vi "SVT Set Swept Sine Propagation Delays.vi"(8 "error in (no error)":errorcluster, 9 "DUT propagation time [ms]":dbl format="%.2f", 10 "device propagation delay [samples]":dbl=1.0 format="%#.1g", 11 "swept sine task in":T1={"source settings"={"AO task name"="", "source"=[]}, "stimulus settings"={"stimulus task name"="", "stimulus"=[]}, "response(s) settings"={"response task name"="", "response"=[]}, "measurement settings"={"AI sampling frequency"=51200.0, "AO sampling frequency"=51200.0, "AI block size"=5120, "AO block Size"=5120, "block duration [ms]"=100.0, "number of AI channels"=0, "device propagation delay [samples]"=1.0, "total propagation time [samples]"=0.0, "DUT propagation time [ms]"=0.0}, "linlog"=enum."linear", "repeat"=enum."off", "frequency list"=[500.0, 515.1515151515151, 530.3030303030303, 545.4545454545454, 560.6060606060605, 575.7575757575756, 590.9090909090908, 606.0606060606059, 621.212121212121, 636.3636363636361, 651.5151515151513, 666.6666666666664, 681.8181818181815, 696.9696969696967, 712.1212121212118, 727.2727272727269, 742.424242424242, 757.5757575757572, 772.7272727272723, 787.8787878787874, 803.0303030303025, 818.1818181818177, 833.3333333333328, 848.4848484848479, 863.6363636363631, 878.7878787878782, 893.9393939393933, 909.0909090909084, 924.2424242424236, 939.3939393939387, 954.5454545454538, 969.696969696969, 984.8484848484841, 999.9999999999992, 1015.1515151515143, 1030.3030303030296, 1045.4545454545448, 1060.60606060606, 1075.7575757575753, 1090.9090909090905, 1106.0606060606058, 1121.212121212121, 1136.3636363636363, 1151.5151515151515, 1166.6666666666667, 1181.818181818182, 1196.9696969696972, 1212.1212121212125, 1227.2727272727277, 1242.424242424243, 1257.5757575757582, 1272.7272727272734, 1287.8787878787887, 1303.030303030304, 1318.1818181818192, 1333.3333333333344, 1348.4848484848496, 1363.6363636363649, 1378.7878787878801, 1393.9393939393954, 1409.0909090909106, 1424.2424242424258, 1439.393939393941, 1454.5454545454563, 1469.6969696969716, 1484.8484848484868, 1500.000000000002, 1515.1515151515173, 1530.3030303030325, 1545.4545454545478, 1560.606060606063, 1575.7575757575783, 1590.9090909090935, 1606.0606060606087, 1621.212121212124, 1636.3636363636392, 1651.5151515151545, 1666.6666666666697, 1681.818181818185, 1696.9696969697002, 1712.1212121212154, 1727.2727272727307, 1742.424242424246, 1757.5757575757611, 1772.7272727272764, 1787.8787878787916, 1803.0303030303069, 1818.181818181822, 1833.3333333333374, 1848.4848484848526, 1863.6363636363678, 1878.787878787883, 1893.9393939393983, 1909.0909090909136, 1924.2424242424288, 1939.393939393944, 1954.5454545454593, 1969.6969696969745, 1984.8484848484898, 2000.000000000005], "amplitude list"=[1.0, 1.0, 1.0, 1.0, 1.0, 1.0, 1.0, 1.0, 1.0, 1.0, 1.0, 1.0, 1.0, 1.0, 1.0, 1.0, 1.0, 1.0, 1.0, 1.0, 1.0, 1.0, 1.0, 1.0, 1.0, 1.0, 1.0, 1.0, 1.0, 1.0, 1.0, 1.0, 1.0, 1.0, 1.0, 1.0, 1.0, 1.0, 1.0, 1.0, 1.0, 1.0, 1.0, 1.0, 1.0, 1.0, 1.0, 1.0, 1.0, 1.0, 1.0, 1.0, 1.0, 1.0, 1.0, 1.0, 1.0, 1.0, 1.0, 1.0, 1.0, 1.0, 1.0, 1.0, 1.0, 1.0, 1.0, 1.0, 1.0, 1.0, 1.0, 1.0, 1.0, 1.0, 1.0, 1.0, 1.0, 1.0, 1.0, 1.0, 1.0, 1.0, 1.0, 1.0, 1.0, 1.0, 1.0, 1.0, 1.0, 1.0, 1.0, 1.0, 1.0, 1.0, 1.0, 1.0, 1.0, 1.0, 1.0, 1.0], "settling time"={"settle time"=0.02, "settle cycles"=5}, "integration time"={"integration time"=0.02, "integration cycles"=5}, "frequencies indices"={"AI freq index"=0, "AO freq index"=0}, "read marks"={"write index"=0, "read index"=0, "freq start index"=0, "freq stop index"=0, "# extracted"=0, "buffer type"=enum."Invalid buffer", "read/write indices"=[{"settle time index"=0, "integration time index"=0}, {"settle time index"=0, "integration time index"=0}, {"settle time index"=0, "integration time index"=0}], "AO index"=0, "AI index"=0, "settled"=FALSE, "integration done"=FALSE}, "harmonic settings"={"maximum THD harmonic"=0, "harmonic mapping"=[], "units"={"THD unit"=enum."%", "nth harmonic unit"=enum."%", "SINAD unit"=enum."dB", "THD+N unit"=enum."dB"}}, "auto resolution settings"={"auto max step"=512, "slow threshold db"=6.0, "fast threshold db"=1.0}, "auto level settings"={"auto level enable"=FALSE, "auto level channel"=6, "ideal ref"=1.0, "max level"=10.0, "ref upper deviation db"=3.0, "ref lower deviation db"=-3.0}, "offset"=0.0, "ramping rate"=0.0, "phase"=0.0, "initialize"=FALSE} {"phase" format="%.2f"; "response(s) settings"."response"."channel info"."pregain" format="%.2f"; "response(s) settings"."response"."channel info"."weighting filter" items=["Linear", "A-weighting", "B-weighting", "C-weighting", "ITU-R 468-4", "Dolby", "CCITT", "C-message", "Wb", "Wc", "Wd", "We", "Wf", "Wh", "Wj", "Wk", "Wm", "AES17 20 kHz lowpass", "AES17 40 kHz lowpass", "AES17 20 kHz highpass", "AES17 40 kHz highpass"]; "response(s) settings"."response"."channel info"."dB reference" format="%^.1e"; "response(s) settings"."response"."channel info"."engineering units" items=["custom..."=0, "V"=1, "A"=21, "C"=30, "pC"=31, "s"=32, "-"=29, "Pa"=2, "N"=20, "g"=3, "m/s^2"=4, "m/s"=5, "m"=6, "mm/s"=12, "mm"=13, "micron/s"=14, "micron"=15, "in/s^2"=7, "in/s"=8, "in"=9, "mil/s"=10, "mil"=11, "rad/s^2"=16, "rad/s"=17, "rad"=18, "deg/s^2"=26, "deg/s"=27, "deg"=28, "RPM"=22, "cycle/s^2"=23, "Hz"=24, "cycle"=25, "strain"=19]; "response(s) settings"."response"."channel info"."sensor sensitivity" format="%#_5f"; "stimulus settings"."stimulus"."channel info"."pregain" format="%.2f"; "stimulus settings"."stimulus"."channel info"."weighting filter" items=["Linear", "A-weighting", "B-weighting", "C-weighting", "ITU-R 468-4", "Dolby", "CCITT", "C-message", "Wb", "Wc", "Wd", "We", "Wf", "Wh", "Wj", "Wk", "Wm", "AES17 20 kHz lowpass", "AES17 40 kHz lowpass", "AES17 20 kHz highpass", "AES17 40 kHz highpass"]; "stimulus settings"."stimulus"."channel info"."dB reference" format="%^.1e"; "stimulus settings"."stimulus"."channel info"."engineering units" items=["custom..."=0, "V"=1, "A"=21, "C"=30, "pC"=31, "s"=32, "-"=29, "Pa"=2, "N"=20, "g"=3, "m/s^2"=4, "m/s"=5, "m"=6, "mm/s"=12, "mm"=13, "micron/s"=14, "micron"=15, "in/s^2"=7, "in/s"=8, "in"=9, "mil/s"=10, "mil"=11, "rad/s^2"=16, "rad/s"=17, "rad"=18, "deg/s^2"=26, "deg/s"=27, "deg"=28, "RPM"=22, "cycle/s^2"=23, "Hz"=24, "cycle"=25, "strain"=19]; "stimulus settings"."stimulus"."channel info"."sensor sensitivity" format="%#_5f"; "ramping rate" format="%.4f"; "offset" format="%.2f"; "auto level settings"."ref lower deviation db" format="%.4f"; "auto level settings"."ref upper deviation db" format="%.4f"; "auto level settings"."max level" format="%.4f"; "auto level settings"."ideal ref" format="%.4f"; "auto resolution settings"."fast threshold db" format="%.4f"; "auto resolution settings"."slow threshold db" format="%.4f"; "harmonic settings"."maximum THD harmonic" max=10 step=1; "integration time"."integration time" format="%.2p"; "settling time"."settle time" format="%.2p"; "amplitude list" format="%.2f"; "frequency list" format="%.2f"; "measurement settings"."DUT propagation time [ms]" format="%.2f"; "measurement settings"."AO sampling frequency" format="%.2f"; "measurement settings"."AI sampling frequency" format="%.2f"}) -> (0 "error out":errorcluster, 3 "swept sine task out":T1={"source settings"={"AO task name"="", "source"=[]}, "stimulus settings"={"stimulus task name"="", "stimulus"=[]}, "response(s) settings"={"response task name"="", "response"=[]}, "measurement settings"={"AI sampling frequency"=51200.0, "AO sampling frequency"=51200.0, "AI block size"=5120, "AO block Size"=5120, "block duration [ms]"=100.0, "number of AI channels"=0, "device propagation delay [samples]"=1.0, "total propagation time [samples]"=0.0, "DUT propagation time [ms]"=0.0}, "linlog"=enum."linear", "repeat"=enum."off", "frequency list"=[500.0, 515.1515151515151, 530.3030303030303, 545.4545454545454, 560.6060606060605, 575.7575757575756, 590.9090909090908, 606.0606060606059, 621.212121212121, 636.3636363636361, 651.5151515151513, 666.6666666666664, 681.8181818181815, 696.9696969696967, 712.1212121212118, 727.2727272727269, 742.424242424242, 757.5757575757572, 772.7272727272723, 787.8787878787874, 803.0303030303025, 818.1818181818177, 833.3333333333328, 848.4848484848479, 863.6363636363631, 878.7878787878782, 893.9393939393933, 909.0909090909084, 924.2424242424236, 939.3939393939387, 954.5454545454538, 969.696969696969, 984.8484848484841, 999.9999999999992, 1015.1515151515143, 1030.3030303030296, 1045.4545454545448, 1060.60606060606, 1075.7575757575753, 1090.9090909090905, 1106.0606060606058, 1121.212121212121, 1136.3636363636363, 1151.5151515151515, 1166.6666666666667, 1181.818181818182, 1196.9696969696972, 1212.1212121212125, 1227.2727272727277, 1242.424242424243, 1257.5757575757582, 1272.7272727272734, 1287.8787878787887, 1303.030303030304, 1318.1818181818192, 1333.3333333333344, 1348.4848484848496, 1363.6363636363649, 1378.7878787878801, 1393.9393939393954, 1409.0909090909106, 1424.2424242424258, 1439.393939393941, 1454.5454545454563, 1469.6969696969716, 1484.8484848484868, 1500.000000000002, 1515.1515151515173, 1530.3030303030325, 1545.4545454545478, 1560.606060606063, 1575.7575757575783, 1590.9090909090935, 1606.0606060606087, 1621.212121212124, 1636.3636363636392, 1651.5151515151545, 1666.6666666666697, 1681.818181818185, 1696.9696969697002, 1712.1212121212154, 1727.2727272727307, 1742.424242424246, 1757.5757575757611, 1772.7272727272764, 1787.8787878787916, 1803.0303030303069, 1818.181818181822, 1833.3333333333374, 1848.4848484848526, 1863.6363636363678, 1878.787878787883, 1893.9393939393983, 1909.0909090909136, 1924.2424242424288, 1939.393939393944, 1954.5454545454593, 1969.6969696969745, 1984.8484848484898, 2000.000000000005], "amplitude list"=[1.0, 1.0, 1.0, 1.0, 1.0, 1.0, 1.0, 1.0, 1.0, 1.0, 1.0, 1.0, 1.0, 1.0, 1.0, 1.0, 1.0, 1.0, 1.0, 1.0, 1.0, 1.0, 1.0, 1.0, 1.0, 1.0, 1.0, 1.0, 1.0, 1.0, 1.0, 1.0, 1.0, 1.0, 1.0, 1.0, 1.0, 1.0, 1.0, 1.0, 1.0, 1.0, 1.0, 1.0, 1.0, 1.0, 1.0, 1.0, 1.0, 1.0, 1.0, 1.0, 1.0, 1.0, 1.0, 1.0, 1.0, 1.0, 1.0, 1.0, 1.0, 1.0, 1.0, 1.0, 1.0, 1.0, 1.0, 1.0, 1.0, 1.0, 1.0, 1.0, 1.0, 1.0, 1.0, 1.0, 1.0, 1.0, 1.0, 1.0, 1.0, 1.0, 1.0, 1.0, 1.0, 1.0, 1.0, 1.0, 1.0, 1.0, 1.0, 1.0, 1.0, 1.0, 1.0, 1.0, 1.0, 1.0, 1.0, 1.0], "settling time"={"settle time"=0.02, "settle cycles"=5}, "integration time"={"integration time"=0.02, "integration cycles"=5}, "frequencies indices"={"AI freq index"=0, "AO freq index"=0}, "read marks"={"write index"=0, "read index"=0, "freq start index"=0, "freq stop index"=100, "# extracted"=0, "buffer type"=enum."Invalid buffer", "read/write indices"=[{"settle time index"=0, "integration time index"=0}, {"settle time index"=0, "integration time index"=0}, {"settle time index"=0, "integration time index"=0}], "AO index"=0, "AI index"=0, "settled"=FALSE, "integration done"=FALSE}, "harmonic settings"={"maximum THD harmonic"=0, "harmonic mapping"=[], "units"={"THD unit"=enum."%", "nth harmonic unit"=enum."%", "SINAD unit"=enum."dB", "THD+N unit"=enum."dB"}}, "auto resolution settings"={"auto max step"=512, "slow threshold db"=6.0, "fast threshold db"=1.0}, "auto level settings"={"auto level enable"=FALSE, "auto level channel"=6, "ideal ref"=1.0, "max level"=10.0, "ref upper deviation db"=3.0, "ref lower deviation db"=-3.0}, "offset"=0.0, "ramping rate"=0.0, "phase"=0.0, "initialize"=FALSE} {"phase" format="%.2f"; "response(s) settings"."response"."channel info"."pregain" format="%.2f"; "response(s) settings"."response"."channel info"."weighting filter" items=["Linear", "A-weighting", "B-weighting", "C-weighting", "ITU-R 468-4", "Dolby", "CCITT", "C-message", "Wb", "Wc", "Wd", "We", "Wf", "Wh", "Wj", "Wk", "Wm", "AES17 20 kHz lowpass", "AES17 40 kHz lowpass", "AES17 20 kHz highpass", "AES17 40 kHz highpass"]; "response(s) settings"."response"."channel info"."dB reference" format="%^.1e"; "response(s) settings"."response"."channel info"."engineering units" items=["custom..."=0, "V"=1, "A"=21, "C"=30, "pC"=31, "s"=32, "-"=29, "Pa"=2, "N"=20, "g"=3, "m/s^2"=4, "m/s"=5, "m"=6, "mm/s"=12, "mm"=13, "micron/s"=14, "micron"=15, "in/s^2"=7, "in/s"=8, "in"=9, "mil/s"=10, "mil"=11, "rad/s^2"=16, "rad/s"=17, "rad"=18, "deg/s^2"=26, "deg/s"=27, "deg"=28, "RPM"=22, "cycle/s^2"=23, "Hz"=24, "cycle"=25, "strain"=19]; "response(s) settings"."response"."channel info"."sensor sensitivity" format="%#_5f"; "stimulus settings"."stimulus"."channel info"."pregain" format="%.2f"; "stimulus settings"."stimulus"."channel info"."weighting filter" items=["Linear", "A-weighting", "B-weighting", "C-weighting", "ITU-R 468-4", "Dolby", "CCITT", "C-message", "Wb", "Wc", "Wd", "We", "Wf", "Wh", "Wj", "Wk", "Wm", "AES17 20 kHz lowpass", "AES17 40 kHz lowpass", "AES17 20 kHz highpass", "AES17 40 kHz highpass"]; "stimulus settings"."stimulus"."channel info"."dB reference" format="%^.1e"; "stimulus settings"."stimulus"."channel info"."engineering units" items=["custom..."=0, "V"=1, "A"=21, "C"=30, "pC"=31, "s"=32, "-"=29, "Pa"=2, "N"=20, "g"=3, "m/s^2"=4, "m/s"=5, "m"=6, "mm/s"=12, "mm"=13, "micron/s"=14, "micron"=15, "in/s^2"=7, "in/s"=8, "in"=9, "mil/s"=10, "mil"=11, "rad/s^2"=16, "rad/s"=17, "rad"=18, "deg/s^2"=26, "deg/s"=27, "deg"=28, "RPM"=22, "cycle/s^2"=23, "Hz"=24, "cycle"=25, "strain"=19]; "stimulus settings"."stimulus"."channel info"."sensor sensitivity" format="%#_5f"; "ramping rate" format="%.4f"; "offset" format="%.2f"; "auto level settings"."ref lower deviation db" format="%.4f"; "auto level settings"."ref upper deviation db" format="%.4f"; "auto level settings"."max level" format="%.4f"; "auto level settings"."ideal ref" format="%.4f"; "auto resolution settings"."fast threshold db" format="%.4f"; "auto resolution settings"."slow threshold db" format="%.4f"; "harmonic settings"."maximum THD harmonic" max=10 step=1; "integration time"."integration time" format="%.2p"; "settling time"."settle time" format="%.2p"; "amplitude list" format="%.2f"; "frequency list" format="%.2f"; "measurement settings"."DUT propagation time [ms]" format="%.2f"; "measurement settings"."AO sampling frequency" format="%.2f"; "measurement settings"."AI sampling frequency" format="%.2f"})   [LabVIEW 2017, in "SoundVib_SweptSine.lvlib"]
doc: "Sets the propagation time, expressed in number of samples, introduced by the data acquisition board used to perform the swept-sine measurement and the propagation time, expressed in milliseconds, introduced by the device under test (DUT)."
uses:
  <vilib>/addons/Sound and Vibration/svt_Swept Sine/SoundVib_SweptSine.lvlib
  <vilib>/addons/Sound and Vibration/svt_Swept Sine/subVIs/sv_Swept Sine Task.ctl
  <vilib>/addons/_NISVFA/_Shared subVIs/Controls/svc_Channel Info.ctl
  <vilib>/addons/_NISVFA/_Shared subVIs/Controls/svc_Engineering Units Text Ring.ctl
  <vilib>/addons/_NISVFA/_Shared subVIs/Controls/svc_Weighting Filter Text Ring.ctl
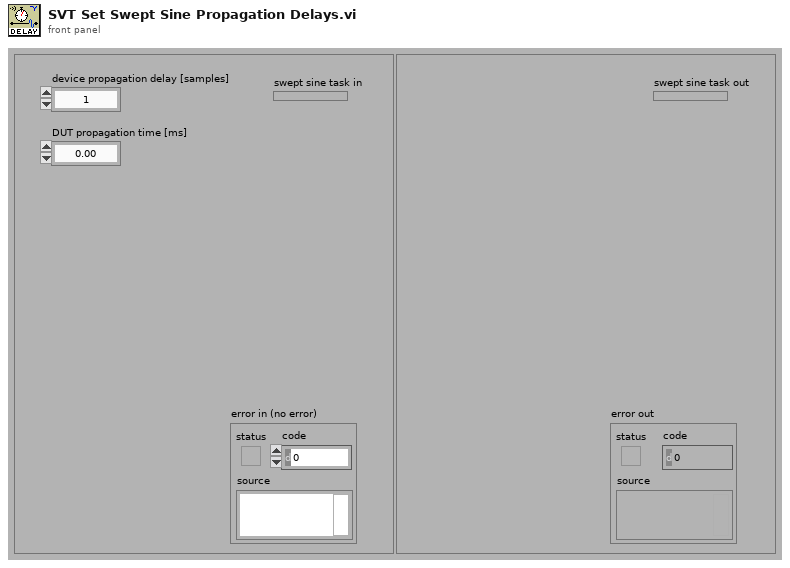
[diagram p1: front panel]
types:
  T1 = typedef "SoundVib_SweptSine.lvlib/sv_Swept Sine Task.ctl" = cluster{"source settings":cluster{"AO task name":refnum<k21>, "source":cluster{"AO physical channel":tag}[]}, "stimulus settings":cluster{"stimulus task name":refnum<k21>, "stimulus":cluster{"stimulus physical channel":tag, "channel info":T2}[]}, "response(s) settings":cluster{"response task name":refnum<k21>, "response":cluster{"response physical channel":tag, "channel info":T2}[]}, "measurement settings":cluster{"AI sampling frequency":dbl, "AO sampling frequency":dbl, "AI block size":i32, "AO block Size":i32, "block duration [ms]":dbl, "number of AI channels":i32, "device propagation delay [samples]":dbl, "total propagation time [samples]":dbl, "DUT propagation time [ms]":dbl}, "linlog":enum16{"linear", "log"}, "repeat":enum16{"off", "on"}, "frequency list":dbl[], "amplitude list":dbl[], "settling time":cluster{"settle time":dbl, "settle cycles":i32}, "integration time":cluster{"integration time":dbl, "integration cycles":i32}, "frequencies indices":cluster{"AI freq index":i32, "AO freq index":i32}, "read marks":cluster{"write index":u32, "read index":u32, "freq start index":u32, "freq stop index":u32, "# extracted":u32, "buffer type":enum16{"Invalid buffer", "Intermediate buffer", "Final buffer"}, "read/write indices":cluster{"settle time index":u32, "integration time index":u32}[], "AO index":i32, "AI index":i32, "settled":bool, "integration done":bool}, "harmonic settings":cluster{"maximum THD harmonic":u32, "harmonic mapping":u32[], "units":cluster{"THD unit":enum16{"dB", "%"}, "nth harmonic unit":enum16{"dB", "%"}, "SINAD unit":enum16{"dB", "%"}, "THD+N unit":enum16{"dB", "%"}}}, "auto resolution settings":cluster{"auto max step":i32, "slow threshold db":dbl, "fast threshold db":dbl}, "auto level settings":cluster{"auto level enable":bool, "auto level channel":u8, "ideal ref":sgl, "max level":sgl, "ref upper deviation db":sgl, "ref lower deviation db":sgl}, "offset":dbl, "ramping rate":dbl, "phase":dbl, "initialize":bool}
  T2 = typedef "svc_Channel Info.ctl" = cluster{"sensor sensitivity":dbl, "engineering units":T3, "dB reference":dbl, "custom label":string, "weighting filter":T4, "pregain":dbl}
  T3 = typedef "svc_Engineering Units Text Ring.ctl" = u16
  T4 = typedef "svc_Weighting Filter Text Ring.ctl" = u16
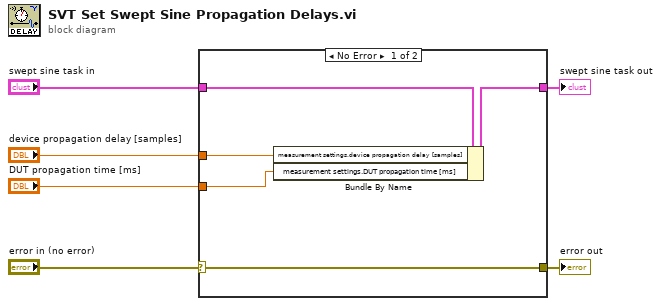
[diagram p0: block diagram]
diagram:
  n1 = case shown="No Error" "error in (no error)" {
    selector: "error in (no error)" -> [w8 w13]
    tunnel: "DUT propagation time [ms]" -> [w7 _]
    tunnel: [w8 w13] -> w2
    tunnel: "swept sine task in" -> [w11 w12]
    tunnel: [w10 w12] -> w3
    tunnel: "device propagation delay [samples]" -> [w9 _]
    frame No Error {
      n2 = Bundle By Name(cluster=w11, "measurement settings.device propagation delay [samples]"=w9, "measurement settings.DUT propagation time [ms]"=w7) -> (w10:T1)
    }
    frame Error {
    }
  }
  "swept sine task out" <- w3
  "error out" <- w2
